vi "DAQmx - Get Accele Task Chan Names_SubVIs-某型振动实验台测试系统.vi"(1 "Accele Task":T1[](array[typedef])) -> (0 "Chan Names":string[](array[string]))   [LabVIEW 2011]
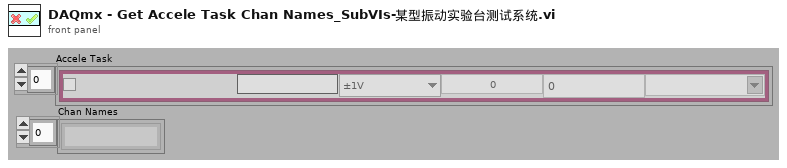
[diagram p1: front panel]
types:
  T1 = typedef "Acceleration Channel Config_Ctrls-某型振动实验台测试系统.ctl" = cluster{"Enable":bool, "Name":string, "range":enum16{"±1V", "±5V"}, "SensValue":dbl, "PhysicalName":string, "off":dbl, "Sensunits":string}
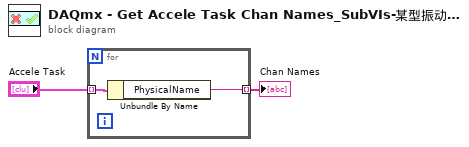
[diagram p0: block diagram]
diagram:
  n1 = for {
    tunnel: "Accele Task" -> [w4] mode=indexing
    tunnel: [w3] -> w1 mode=indexing
    n2 = Unbundle By Name(w4) -> ("PhysicalName"=w3:string)
  }
  "Chan Names" <- w1
